vi "SnapAndCalibration.vi"(8 "error in (no error)":errorcluster, 11 "Value":u16) -> (0 "error out":errorcluster, 3 "Image Dst Out":T1)   [LabVIEW 2019]
uses:
  <vilib>/vision/Image Controls.llb/IMAQ Image.ctl
  iVision/Controls/Parameter.ctl
  <vilib>/vision/NI_Vision_Development_Module.lvlib
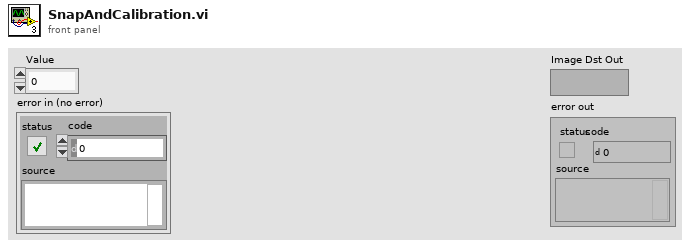
[diagram p1: front panel]
types:
  T1 = typedef "IMAQ Image.ctl" = refnum<image>
  T2 = typedef "Parameter.ctl" = enum16{"Initialize", "Write", "Read", "WriteAll", "Save", "Load"}
  T3 = enum16{"Init", "Grab", "Get All", "Close", "Set Camera"}
  T4 = typedef "ParameterData.ctl" = cluster{"Rotate Angle":dbl, "Rotate?":bool, "Calibration File Path":string, "Cal?":bool}
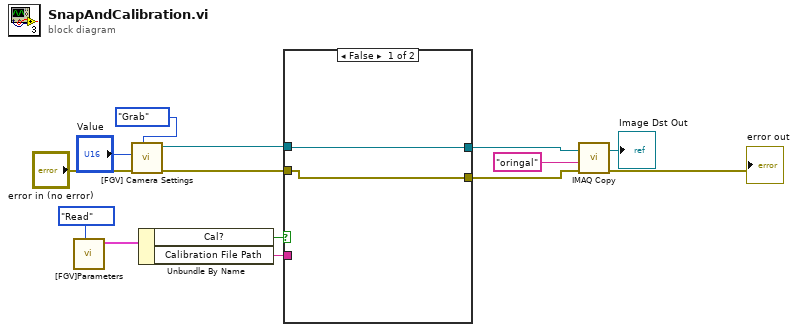
[diagram p0: block diagram]
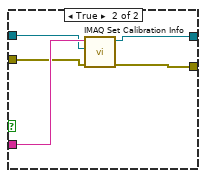
[diagram p2: hidden frame]
diagram:
  n1 = call "[FGV]Parameters.vi"("Parameter"=Parameter."Read") -> ("ParameterData Out"=w10:T4)  [unwired: 9 in, 1 out]
  n2 = call "[FGV] Camera Settings.vi"("Action"=T3."Grab", "error in (no error)"="error in (no error)", "Value"="Value") -> ("error out"=w4:errorcluster, "Image Out"=w12:T1)  [unwired: 6 in, 1 out]
  n3 = Unbundle By Name(w10) -> ("Cal?"=w11:bool, "Calibration File Path"=w13:string)
  n4 = case shown="False" w11 {
    tunnel: w12 -> [w16 w20]
    tunnel: w13 -> [_ w21]
    tunnel: [w16 w19] -> w14
    tunnel: w4 -> [w15 w18]
    tunnel: [w15 w17] -> w3
    frame False {
    }
    frame True {
      n5 = call "IMAQ Set Calibration Info"("error in (no error)"=w18, "Image Dst"=w20, "Image Src"=w21) -> ("error out"=w17:errorcluster, "Calibrated Image"=w19:T1)  [unwired: 7 in]
    }
  }
  n6 = call "IMAQ Copy"("error in (no error)"=w3, "Image Dst"="oringal" ("Image Name"), "Image Src"=w14) -> ("error out"=→"error out":errorcluster, "Image Dst Out"=→"Image Dst Out":T1)  [unwired: 3 in]
